vi "Robot Drive Manual.vi"(0 "Joystick0DevRef":T2={"Device"=enum."USB 1"}, 1 "RobotDriveDevRef":T4={"DevStatus"={"status"=FALSE, "code"=0, "source"=""}, "Motors[]"=[], "Square Inputs"=FALSE, "Max Output"=1.0}, 5 "Joystick1DevRef":T2={"Device"=enum."USB 1"}, 7 "Call Context":T1, 9 "Controller Mode":enum16{"X-Box Controller", "Joysticks"}(ring), 11 "Drive Mode":enum16{"Tank Drive", "Arcade Drive"}(ring), 12 "dt":dbl) -> (6 "Motor Values":dbl[](array[numeric]))   [LabVIEW 2016]
uses:
  <vilib>/Rock Robotics/WPI/RobotDrive/WPI_RobotDriveDevRef.ctl
  <vilib>/Rock Robotics/WPI/MotorControl/WPI_MotorControlDeviceRef.ctl
  <vilib>/Rock Robotics/WPI/MotorControl/WPI_MotorControlType.ctl
  <vilib>/Rock Robotics/SystemInterfaces/DIO/FPGA_DIOPWMChannel.ctl
  <vilib>/Rock Robotics/WPI/PWM/WPI_PWMDeadband.ctl
  <vilib>/Rock Robotics/WPI/Joystick/WPI_JoystickDevRef.ctl
  <vilib>/Rock Robotics/WPI/Joystick/WPI_JoystickDeviceEnum.ctl
  <vilib>/Rock Robotics/WPI/DriverStation/WPI_DriverStationDerivedRobotMode.ctl
  <vilib>/Rock Robotics/Network Tables/NT Read Boolean.vi
  Robot Global Data.vi
  <vilib>/Rock Robotics/Network Tables/NT Read Number.vi
  <vilib>/Rock Robotics/Network Tables/NT Write Numeric Array.vi
panel:
  in  "Axes (Joystick 1)":dbl[](array[numeric])
  in  "Axes (Joystick 0)":dbl[](array[numeric])
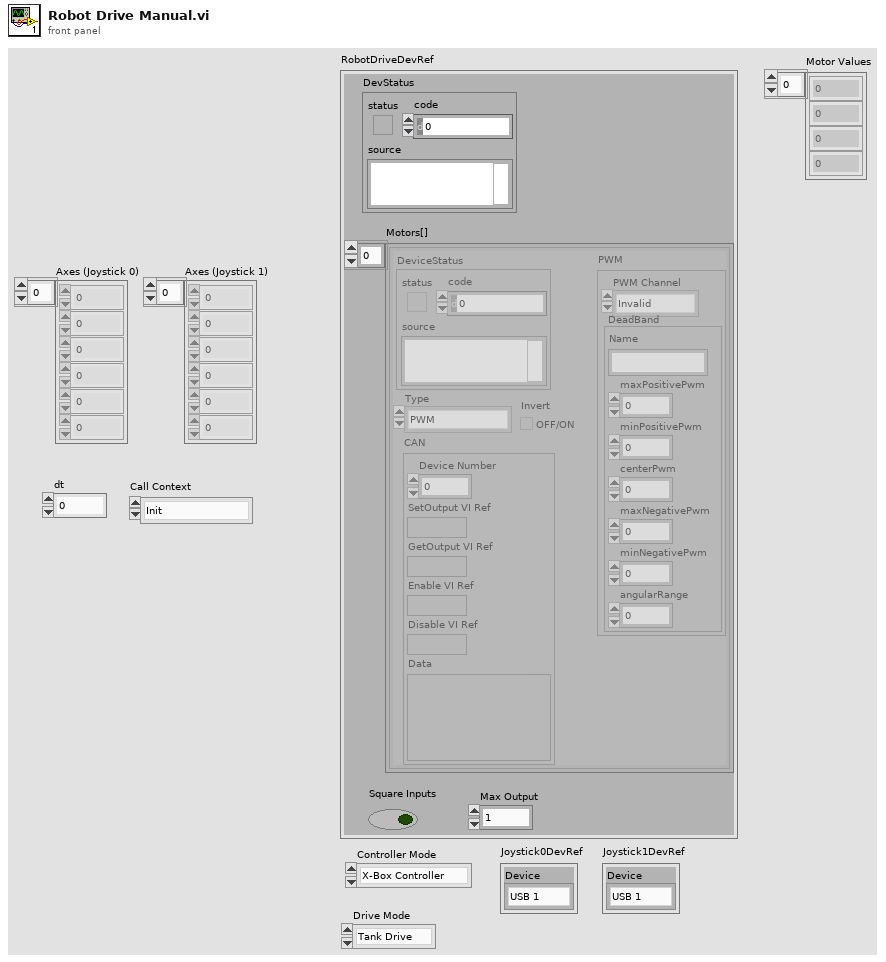
[diagram p1: front panel]
types:
  T1 = typedef "WPI_DriverStationDerivedRobotMode.ctl" = enum16{"Init", "Execute", "Stop"}
  T2 = typedef "WPI_JoystickDevRef.ctl" = cluster{"Device":T3}
  T3 = typedef "WPI_JoystickDeviceEnum.ctl" = enum16{"USB 0", "USB 1", "USB 2", "USB 3", "USB 4", "USB 5"}
  T4 = typedef "WPI_RobotDriveDevRef.ctl" = cluster{"DevStatus":errorcluster, "Motors[]":T5[], "Square Inputs":bool, "Max Output":dbl}
  T5 = typedef "WPI_MotorControlDeviceRef.ctl" = cluster{"DeviceStatus":errorcluster, "Type":T6, "PWM":cluster{"PWM Channel":T7, "DeadBand":T8}, "CAN":cluster{"Device Number":u8, "SetOutput VI Ref":variant, "GetOutput VI Ref":variant, "Enable VI Ref":variant, "Disable VI Ref":variant, "Data":variant}, "Invert":bool}
  T6 = typedef "WPI_MotorControlType.ctl" = enum16{"PWM", "CAN"}
  T7 = typedef "FPGA_DIOPWMChannel.ctl" = enum8{"PWM 0", "PWM 1", "PWM 2", "PWM 3", "PWM 4", "PWM 5", "PWM 6", "PWM 7", "PWM 8", "PWM 9", "PWM MXP 0", "PWM MXP 1", "PWM MXP 2", "PWM MXP 3", "PWM MXP 4", "PWM MXP 5", "PWM MXP 6", "PWM MXP 7", "PWM MXP 8", "PWM MXP 9", "Invalid"}
  T8 = typedef "WPI_PWMDeadband.ctl" = cluster{"Name":string, "maxPositivePwm":i32, "minPositivePwm":i32, "centerPwm":i32, "maxNegativePwm":i32, "minNegativePwm":i32, "angularRange":u16}
  T9 = cluster{"Current Gear":enum16{"Low", "High"}, "Gear Shift State":enum16{"Low", "Shifting", "High"}}
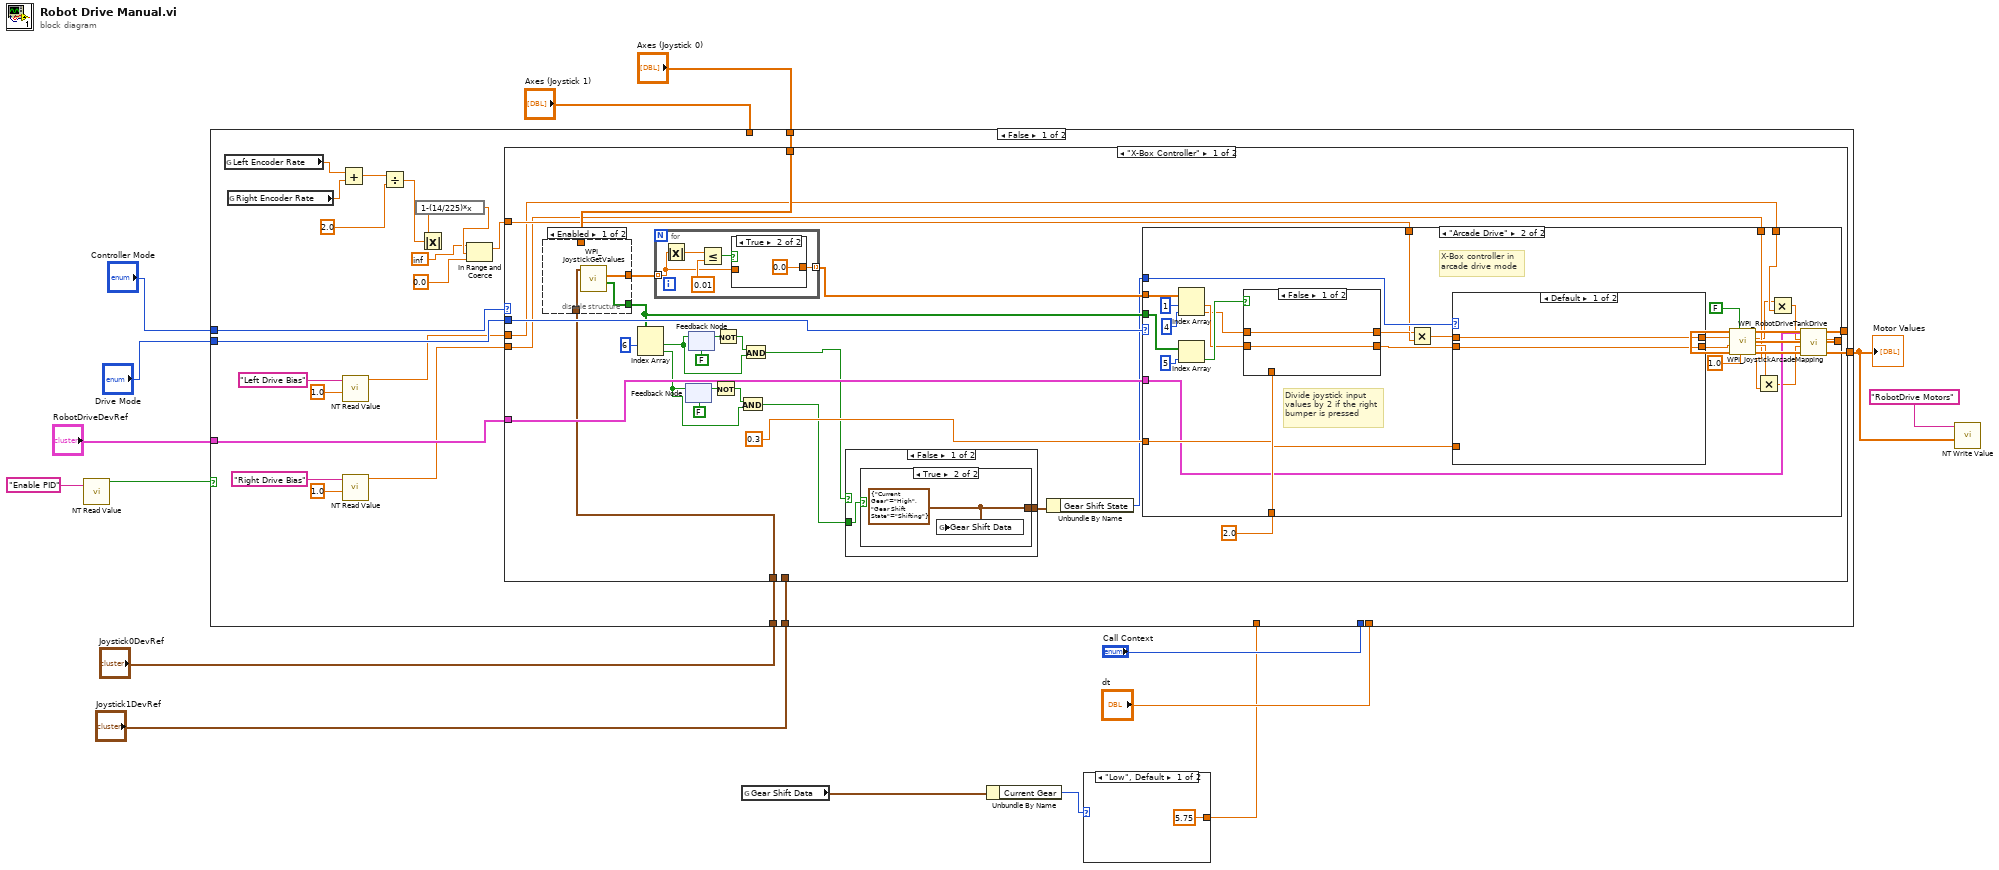
[diagram p0: block diagram]
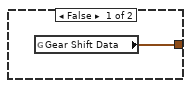
[diagram p2: hidden frame]
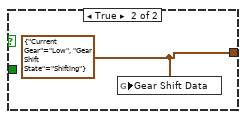
[diagram p3: hidden frame]
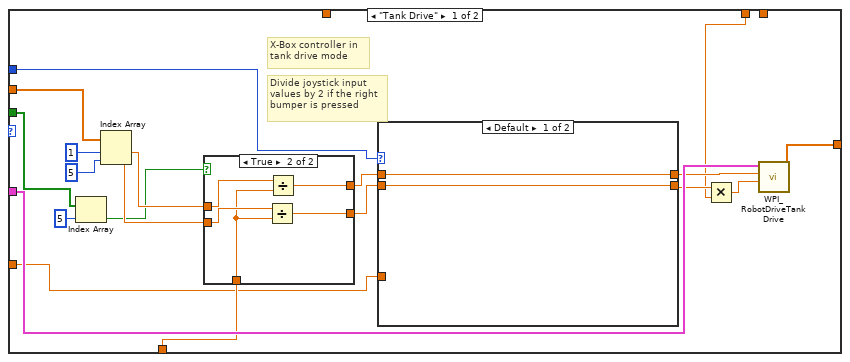
[diagram p4: hidden frame]
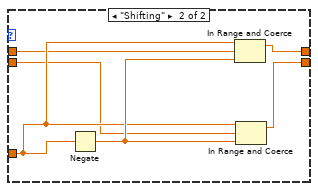
[diagram p5: hidden frame]
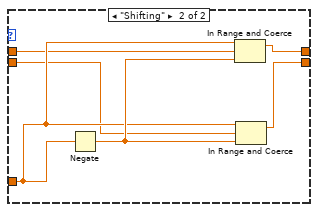
[diagram p7: hidden frame]
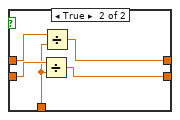
[diagram p8: hidden frame]
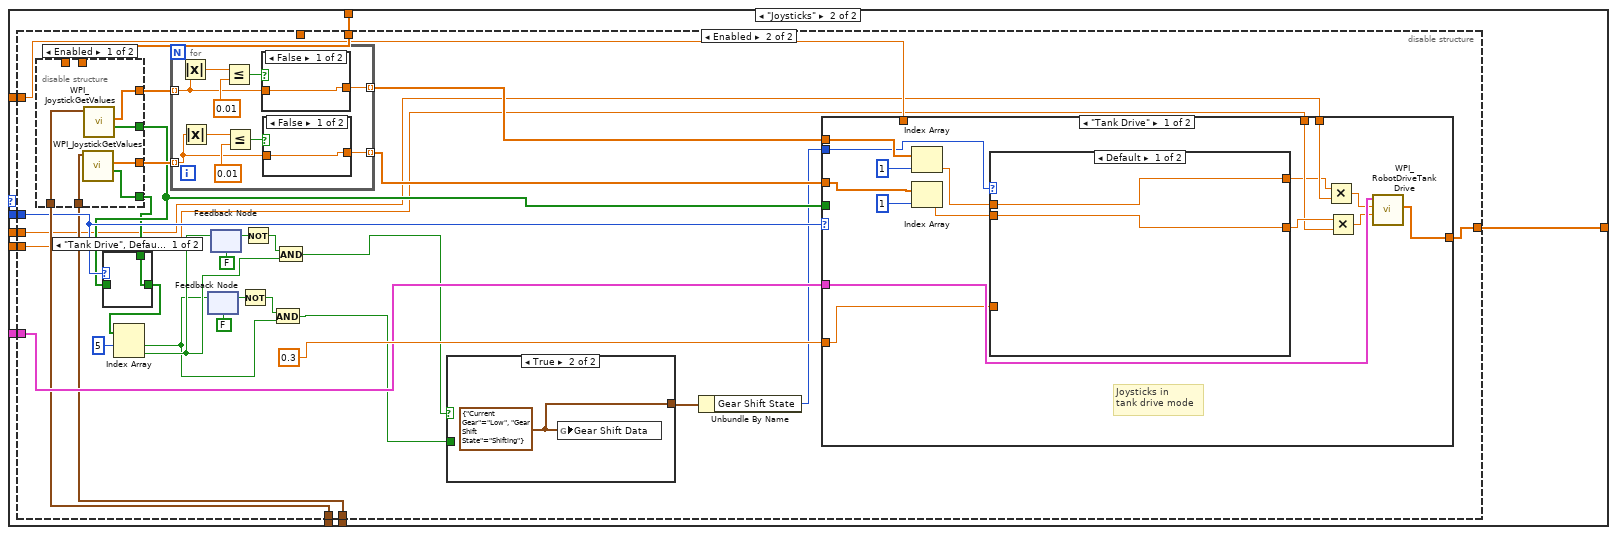
[diagram p11: hidden frame]
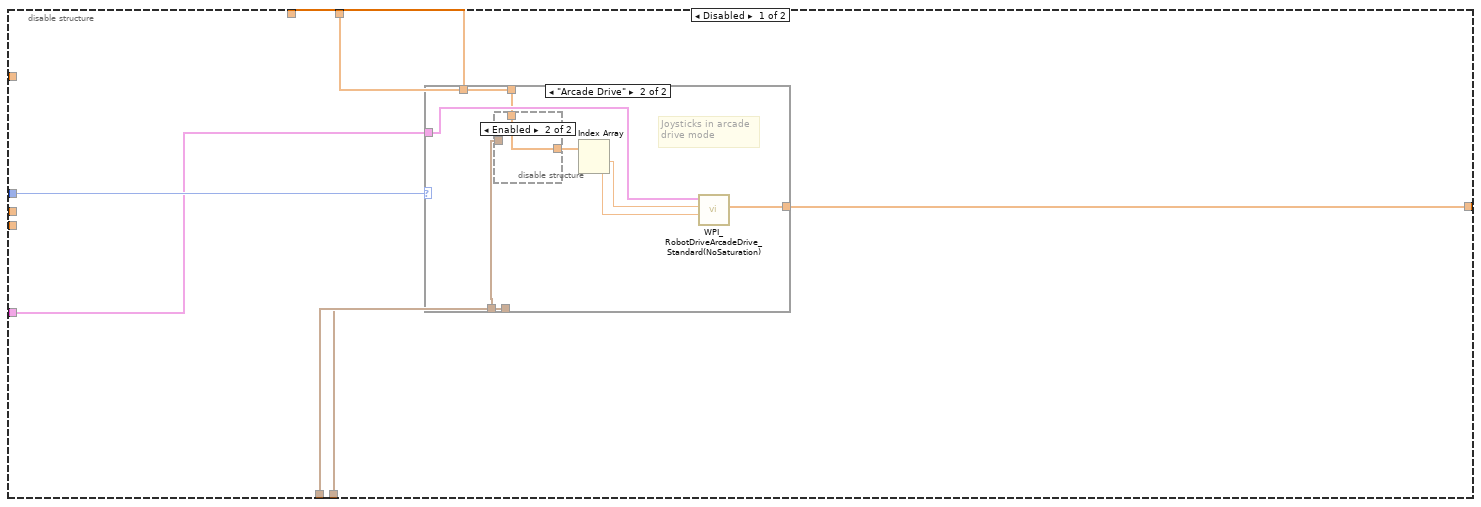
[diagram p12: hidden frame]
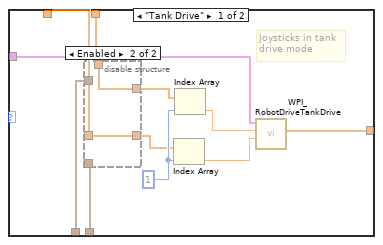
[diagram p13: hidden frame]
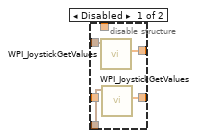
[diagram p14: hidden frame]
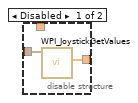
[diagram p15: hidden frame]
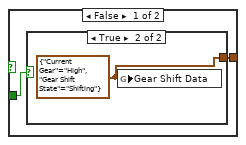
[diagram p16: hidden frame]
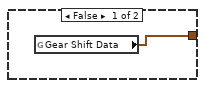
[diagram p17: hidden frame]
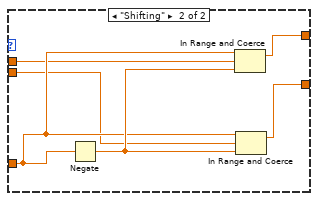
[diagram p18: hidden frame]
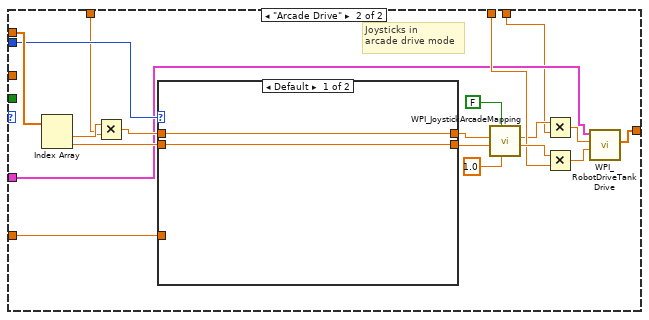
[diagram p19: hidden frame]
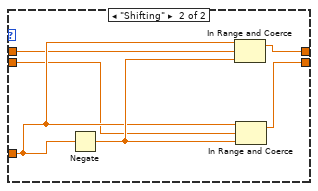
[diagram p20: hidden frame]
diagram:
  n1 = call-poly <vilib>:"NT Read Value.vi"("Name"="Enable PID") -> ("Boolean"=w1:bool)  [unwired: 9 in, 1 out]
  n2 = global read "Robot Global Data.vi" "Gear Shift Data"() -> (w5:T9)
  n3 = Unbundle By Name(w5) -> ("Current Gear"=w4:enum16{"Low", "High"})
  n4 = case shown="\"Low\", Default" w4 {
    tunnel: [5.75 14.75] -> w3
    frame "Low", Default {
    }
    frame "High" {
    }
  }
  n5 = case shown="False" w1 {
    tunnel: "Controller Mode" -> [w41 w324]
    tunnel: "Drive Mode" -> [w40 w323]
    tunnel: "RobotDriveDevRef" -> [w39 w322]
    tunnel: "Joystick0DevRef" -> [w38 w321]
    tunnel: "Joystick1DevRef" -> [w35 w320]
    tunnel: "Axes (Joystick 0)" -> [w37 w319]
    tunnel: "Axes (Joystick 1)" -> [_ w318]
    tunnel: [w36 w317] -> w8
    tunnel: "Call Context" -> [_ w316]
    tunnel: "dt" -> [_ w315]
    tunnel: w3 -> [_ w314]
    frame False {
      n6 = global read "Robot Global Data.vi" "Left Encoder Rate"() -> (w34:dbl)
      n7 = global read "Robot Global Data.vi" "Right Encoder Rate"() -> (w33:dbl)
      n8 = Add(x=w34, y=w33) -> (x+y=w32:dbl)
      n9 = call-poly <vilib>:"NT Read Value.vi"("Default Value"=1.0, "Name"="Left Drive Bias") -> ("Numeric"=w19:dbl)  [unwired: 8 in, 1 out]
      n10 = call-poly <vilib>:"NT Read Value.vi"("Default Value"=1.0, "Name"="Right Drive Bias") -> ("Numeric"=w23:dbl)  [unwired: 8 in, 1 out]
      n11 = Divide(x=w32, y=2.0) -> (x/y=w29:dbl)
      n12 = Absolute Value(x=w29) -> (abs(x)=w30:dbl)
      n13 = expression code="1-(14/225)*x"(w30) -> (w28:dbl)
      n14 = In Range and Coerce(upper limit=inf, x=w28, lower limit=0.0) -> (coerced(x)=w25:dbl)  [unwired: 1 out]
      n15 = case shown="\"X-Box Controller\"" w41 {
        tunnel: w40 -> [w67 w168]
        tunnel: w39 -> [w66 w166]
        tunnel: w38 -> [w64 w167]
        tunnel: [w65 w165] -> w36
        tunnel: w37 -> [w63 w164]
        tunnel: w35 -> [_ w163]
        tunnel: w25 -> [w44 w162]
        tunnel: w23 -> [w43 w161]
        tunnel: w19 -> [w42 w160]
        frame "X-Box Controller" {
          n16 = disable-structure shown="Enabled" {
            disable-tunnel: [w158 w159] -> w51
            disable-tunnel: w64 -> [w157 _]
            disable-tunnel: w63 -> [_ w159]
            disable-tunnel: [w156 _] -> w62
            frame Enabled {
              n17 = call <vilib>:"WPI_JoystickGetValues.vi"("JoystickDevRef"=w157) -> ("Buttons"=w156:bool[], "Axes"=w158:dbl[])  [unwired: 6 in, 3 out]
            }
            frame Disabled {
            }
          }
          n18 = Index Array(array=w62, index #1=6 ("index")) -> (element #1=w57:bool, element #2=w53:bool)  [unwired: 1 in]
          n19 = for {
            tunnel: w51 -> [w149] mode=indexing
            tunnel: [w150] -> w50 mode=indexing
            n20 = Absolute Value(x=w149) -> (abs(x)=w152:dbl)
            n21 = Less Or Equal?(x=w152, y=0.01) -> (x <= y?=w153:bool)
            n22 = case shown="True" w153 {
              tunnel: [w154 0.0] -> w150
              tunnel: w149 -> [w154 _]
              frame False {
              }
              frame True {
              }
            }
          }
          n23 = feedback #1(FALSE) -> (w55:bool)
          n24 = feedback-in #1(w53) -> ()
          n25 = feedback-in #2(w57) -> ()
          n26 = feedback #2(FALSE) -> (w59:bool)
          n27 = Not(x=w55) -> (.not. x?=w54:bool)
          n28 = Not(x=w59) -> (.not. x?=w58:bool)
          n29 = And(x=w54, y=w53) -> (x .and. y?=w47:bool)
          n30 = And(x=w58, y=w57) -> (x .and. y?=w48:bool)
          n31 = case shown="False" w48 {
            tunnel: w47 -> [w69 _]
            tunnel: [w68 w72] -> w46
            frame False {
              n32 = case shown="True" w69 {
                tunnel: [w70 w71] -> w68
                frame False {
                  n33 = global read "Robot Global Data.vi" "Gear Shift Data"() -> (w70:T9)
                }
                frame True {
                  w71 = T9 {"Current Gear"=enum."High", "Gear Shift State"=enum."Shifting"} ("Gear Shift Data")
                  n34 = global write "Robot Global Data.vi" "Gear Shift Data"(w71) -> ()
                }
              }
            }
            frame True {
              w72 = T9 {"Current Gear"=enum."Low", "Gear Shift State"=enum."Shifting"} ("Gear Shift Data")
              n35 = global write "Robot Global Data.vi" "Gear Shift Data"(w72) -> ()
            }
          }
          n36 = Unbundle By Name(w46) -> ("Gear Shift State"=w45:enum16{"Low", "Shifting", "High"})
          n37 = case shown="\"Arcade Drive\"" w67 {
            tunnel: w66 -> [w89 w113]
            tunnel: [w88 w114] -> w65
            tunnel: 2.0 -> [w85 w131]
            tunnel: w50 -> [w82 w130]
            tunnel: w62 -> [w81 w129]
            tunnel: 0.3 ("Left axis value") -> [w78 w126]
            tunnel: w45 -> [w77 w125]
            tunnel: w44 -> [_ w119]
            tunnel: w43 -> [w73 w110]
            tunnel: w42 -> [_ w108]
            frame "Tank Drive" {
              # "Divide joystick input\nvalues by 2 if the right\nbumper is pressed"
              # "X-Box controller in\ntank drive mode"
              n38 = Index Array(array=w81, index=5) -> (element=w83:bool)
              n39 = Index Array(array=w82, index #1=1 ("index"), index #2=5 ("index")) -> (element #1=w87:dbl, element #2=w86:dbl)
              n40 = case shown="True" w83 {
                tunnel: [w101 w106] -> w80
                tunnel: w87 -> [w101 w104]
                tunnel: [w100 w105] -> w79
                tunnel: w86 -> [w100 w103]
                tunnel: w85 -> [_ w102]
                frame False {
                }
                frame True {
                  n41 = Divide(x=w103, y=w102) -> (x/y=w105:dbl)
                  n42 = Divide(x=w104, y=w102) -> (x/y=w106:dbl)
                }
              }
              n43 = case shown="Default" w77 {
                tunnel: [w93 w95] -> w76
                tunnel: w80 -> [w93 w97]
                tunnel: [w92 w94] -> w74
                tunnel: w79 -> [w92 w96]
                tunnel: w78 -> [_ w98]
                frame Default {
                }
                frame "Shifting" {
                  n44 = Negate(x=w98) -> (-x=w99:dbl)
                  n45 = In Range and Coerce(upper limit=w98, x=w97, lower limit=w99) -> (coerced(x)=w95:dbl)  [unwired: 1 out]
                  n46 = In Range and Coerce(upper limit=w98, x=w96, lower limit=w99) -> (coerced(x)=w94:dbl)  [unwired: 1 out]
                }
              }
              n47 = Multiply(x=w74, y=w73) -> (x*y=w75:dbl)
              n48 = call <vilib>:"WPI_RobotDriveTankDrive.vi"("Right axis value"=w75, "Left axis value"=w76, "RobotDriveDevRef"=w89) -> ("Motor Values"=w88:dbl[])  [unwired: 6 in, 2 out]
            }
            frame "Arcade Drive" {
              # "Divide joystick input\nvalues by 2 if the right\nbumper is pressed"
              # "X-Box controller in\narcade drive mode"
              n49 = Index Array(array=w130, index #1=1 ("index"), index #2=4 ("index")) -> (element #1=w123:dbl, element #2=w122:dbl)
              n50 = Index Array(array=w129, index=5) -> (element=w132:bool)
              n51 = case shown="False" w132 {
                tunnel: [w143 w148] -> w120
                tunnel: w122 -> [w143 w146]
                tunnel: [w142 w147] -> w127
                tunnel: w123 -> [w142 w145]
                tunnel: w131 -> [_ w144]
                frame False {
                }
                frame True {
                  n52 = Divide(x=w145, y=w144) -> (x/y=w147:dbl)
                  n53 = Divide(x=w146, y=w144) -> (x/y=w148:dbl)
                }
              }
              n54 = Multiply(x=w119, y=w120) -> (x*y=w121:dbl)
              n55 = case shown="Default" w125 {
                tunnel: [w135 w137] -> w118
                tunnel: w121 -> [w135 w139]
                tunnel: [w134 w136] -> w117
                tunnel: w127 -> [w134 w138]
                tunnel: w126 -> [_ w140]
                frame Default {
                }
                frame "Shifting" {
                  n56 = Negate(x=w140) -> (-x=w141:dbl)
                  n57 = In Range and Coerce(upper limit=w140, x=w139, lower limit=w141) -> (coerced(x)=w137:dbl)  [unwired: 1 out]
                  n58 = In Range and Coerce(upper limit=w140, x=w138, lower limit=w141) -> (coerced(x)=w136:dbl)  [unwired: 1 out]
                }
              }
              n59 = call <vilib>:"WPI_JoystickArcadeMapping.vi"("Max Output"=1.0, "Square Inputs"=FALSE, "Y axis value"=w117, "X axis value"=w118) -> ("Right Motor Value"=w111:dbl, "Left Motor Value"=w107:dbl)  [unwired: 6 in]
              n60 = Multiply(x=w111, y=w110) -> (x*y=w112:dbl)
              n61 = Multiply(x=w107, y=w108) -> (x*y=w109:dbl)
              n62 = call <vilib>:"WPI_RobotDriveTankDrive.vi"("Right axis value"=w112, "Left axis value"=w109, "RobotDriveDevRef"=w113) -> ("Motor Values"=w114:dbl[])  [unwired: 6 in, 2 out]
            }
          }
        }
        frame "Joysticks" {
          n63 = disable-structure shown="Enabled" {
            disable-tunnel: w168 -> [w175 w217]
            disable-tunnel: w167 -> [w174 w220]
            disable-tunnel: w163 -> [w173 w210]
            disable-tunnel: w166 -> [w172 w222]
            disable-tunnel: [w171 w213] -> w165
            disable-tunnel: w164 -> [w170 w221]
            disable-tunnel: _ -> [w169 _]
            disable-tunnel: w162 -> [_ w205]
            disable-tunnel: w161 -> [_ w204]
            disable-tunnel: w160 -> [_ w203]
            frame Disabled {
              n64 = case shown="\"Arcade Drive\"" w175 {
                tunnel: w174 -> [w186 w195]
                tunnel: w173 -> [w185 _]
                tunnel: w172 -> [w181 w196]
                tunnel: [w178 w194] -> w171
                tunnel: w170 -> [w177 w193]
                tunnel: w169 -> [w176 _]
                frame "Tank Drive" {
                  w184 = 1
                  # "Joysticks in tank\ndrive mode"
                  n65 = disable-structure shown="Enabled" {
                    disable-tunnel: w186 -> [w190 _]
                    disable-tunnel: w185 -> [w189 _]
                    disable-tunnel: [w188 w192] -> w183
                    disable-tunnel: [w187 w191] -> w182
                    disable-tunnel: w177 -> [_ w192]
                    disable-tunnel: w176 -> [_ w191]
                    frame Disabled {
                      n66 = call <vilib>:"WPI_JoystickGetValues.vi"("JoystickDevRef"=w190) -> ("Axes"=w188:dbl[])  [unwired: 6 in, 4 out]
                      n67 = call <vilib>:"WPI_JoystickGetValues.vi"("JoystickDevRef"=w189) -> ("Axes"=w187:dbl[])  [unwired: 6 in, 4 out]
                    }
                    frame Enabled {
                    }
                  }
                  n68 = Index Array(array=w182, index=w184) -> (element=w179:dbl)
                  n69 = Index Array(array=w183, index=w184) -> (element=w180:dbl)
                  n70 = call <vilib>:"WPI_RobotDriveTankDrive.vi"("Right axis value"=w179, "Left axis value"=w180, "RobotDriveDevRef"=w181) -> ("Motor Values"=w178:dbl[])  [unwired: 6 in, 2 out]
                }
                frame "Arcade Drive" {
                  # "Joysticks in arcade\ndrive mode"
                  n71 = disable-structure shown="Enabled" {
                    disable-tunnel: [w201 w202] -> w199
                    disable-tunnel: w195 -> [w200 _]
                    disable-tunnel: w193 -> [_ w202]
                    frame Disabled {
                      n72 = call <vilib>:"WPI_JoystickGetValues.vi"("JoystickDevRef"=w200) -> ("Axes"=w201:dbl[])  [unwired: 6 in, 4 out]
                    }
                    frame Enabled {
                    }
                  }
                  n73 = Index Array(array=w199) -> (element #1=w198:dbl, element #2=w197:dbl)  [unwired: 2 in]
                  n74 = call <vilib>:"WPI_RobotDriveArcadeDrive_Standard(NoSaturation).vi"("Y axis value"=w197, "X axis value"=w198, "RobotDriveDevRef"=w196) -> ("Motor Values"=w194:dbl[])  [unwired: 1 in, 7 out]
                }
              }
            }
            frame Enabled {
              n75 = disable-structure shown="Enabled" {
                disable-tunnel: [w310 w311] -> w231
                disable-tunnel: w221 -> [_ w312]
                disable-tunnel: [w309 _] -> w214
                disable-tunnel: w220 -> [w308 _]
                disable-tunnel: [w307 w312] -> w219
                disable-tunnel: _ -> [_ w311]
                disable-tunnel: [w306 _] -> w216
                disable-tunnel: w210 -> [w305 _]
                frame Enabled {
                  n76 = call <vilib>:"WPI_JoystickGetValues.vi"("JoystickDevRef"=w305) -> ("Buttons"=w309:bool[], "Axes"=w310:dbl[])  [unwired: 6 in, 3 out]
                  n77 = call <vilib>:"WPI_JoystickGetValues.vi"("JoystickDevRef"=w308) -> ("Buttons"=w306:bool[], "Axes"=w307:dbl[])  [unwired: 6 in, 3 out]
                }
                frame Disabled {
                }
              }
              n78 = case shown="\"Tank Drive\", Default" w217 {
                tunnel: w216 -> [_ w290]
                tunnel: [w289 w290] -> w215
                tunnel: w214 -> [w289 _]
                frame "Tank Drive", Default {
                }
                frame "Arcade Drive" {
                }
              }
              n79 = Index Array(array=w215, index #1=5 ("index")) -> (element #1=w211:bool, element #2=w212:bool)  [unwired: 1 in]
              n80 = for {
                tunnel: w231 -> [w296] mode=indexing
                tunnel: [w297] -> w232 mode=indexing
                tunnel: w219 -> [w291] mode=indexing
                tunnel: [w292] -> w218 mode=indexing
                n81 = Absolute Value(x=w291) -> (abs(x)=w294:dbl)
                n82 = Absolute Value(x=w296) -> (abs(x)=w299:dbl)
                n83 = Less Or Equal?(x=w294, y=0.01) -> (x <= y?=w295:bool)
                n84 = Less Or Equal?(x=w299, y=0.01) -> (x <= y?=w300:bool)
                n85 = case shown="False" w295 {
                  tunnel: [w301 0.0] -> w292
                  tunnel: w291 -> [w301 _]
                  frame False {
                  }
                  frame True {
                  }
                }
                n86 = case shown="False" w300 {
                  tunnel: [w303 0.0] -> w297
                  tunnel: w296 -> [w303 _]
                  frame False {
                  }
                  frame True {
                  }
                }
              }
              n87 = feedback #3(FALSE) -> (w228:bool)
              n88 = feedback-in #3(w211) -> ()
              n89 = feedback #4(FALSE) -> (w225:bool)
              n90 = feedback-in #4(w212) -> ()
              n91 = Not(x=w228) -> (.not. x?=w229:bool)
              n92 = Not(x=w225) -> (.not. x?=w226:bool)
              n93 = And(x=w229, y=w211) -> (x .and. y?=w208:bool)
              n94 = And(x=w226, y=w212) -> (x .and. y?=w209:bool)
              n95 = case shown="True" w209 {
                tunnel: w208 -> [w234 _]
                tunnel: [w233 w237] -> w207
                frame False {
                  n96 = case shown="True" w234 {
                    tunnel: [w235 w236] -> w233
                    frame False {
                      n97 = global read "Robot Global Data.vi" "Gear Shift Data"() -> (w235:T9)
                    }
                    frame True {
                      w236 = T9 {"Current Gear"=enum."High", "Gear Shift State"=enum."Shifting"} ("Gear Shift Data")
                      n98 = global write "Robot Global Data.vi" "Gear Shift Data"(w236) -> ()
                    }
                  }
                }
                frame True {
                  w237 = T9 {"Current Gear"=enum."Low", "Gear Shift State"=enum."Shifting"} ("Gear Shift Data")
                  n99 = global write "Robot Global Data.vi" "Gear Shift Data"(w237) -> ()
                }
              }
              n100 = Unbundle By Name(w207) -> ("Gear Shift State"=w206:enum16{"Low", "Shifting", "High"})
              n101 = case shown="\"Tank Drive\"" w217 {
                tunnel: w222 -> [w252 w265]
                tunnel: [w251 w268] -> w213
                tunnel: w232 -> [w248 _]
                tunnel: w216 -> [_ _]
                tunnel: w218 -> [w249 w280]
                tunnel: 0.3 ("Left axis value") -> [w245 w278]
                tunnel: w206 -> [w244 w277]
                tunnel: w205 -> [_ w274]
                tunnel: w204 -> [w241 w266]
                tunnel: w203 -> [w239 w263]
                frame "Tank Drive" {
                  # "Joysticks in\ntank drive mode"
                  n102 = Index Array(array=w249, index=1) -> (element=w247:dbl)
                  n103 = Index Array(array=w248, index=1) -> (element=w246:dbl)
                  n104 = case shown="Default" w244 {
                    tunnel: [w255 w257] -> w238
                    tunnel: w247 -> [w255 w259]
                    tunnel: [w254 w256] -> w242
                    tunnel: w246 -> [w254 w258]
                    tunnel: w245 -> [_ w260]
                    frame Default {
                    }
                    frame "Shifting" {
                      n105 = Negate(x=w260) -> (-x=w261:dbl)
                      n106 = In Range and Coerce(upper limit=w260, x=w259, lower limit=w261) -> (coerced(x)=w257:dbl)  [unwired: 1 out]
                      n107 = In Range and Coerce(upper limit=w260, x=w258, lower limit=w261) -> (coerced(x)=w256:dbl)  [unwired: 1 out]
                    }
                  }
                  n108 = Multiply(x=w238, y=w239) -> (x*y=w240:dbl)
                  n109 = Multiply(x=w242, y=w241) -> (x*y=w243:dbl)
                  n110 = call <vilib>:"WPI_RobotDriveTankDrive.vi"("Right axis value"=w243, "Left axis value"=w240, "RobotDriveDevRef"=w252) -> ("Motor Values"=w251:dbl[])  [unwired: 6 in, 2 out]
                }
                frame "Arcade Drive" {
                  # "Joysticks in\narcade drive mode"
                  n111 = Index Array(array=w280) -> (element #1=w275:dbl, element #2=w279:dbl)  [unwired: 2 in]
                  n112 = Multiply(x=w275, y=w274) -> (x*y=w276:dbl)
                  n113 = case shown="Default" w277 {
                    tunnel: [w282 w284] -> w273
                    tunnel: w276 -> [w282 w286]
                    tunnel: [w281 w283] -> w272
                    tunnel: w279 -> [w281 w285]
                    tunnel: w278 -> [_ w287]
                    frame Default {
                    }
                    frame "Shifting" {
                      n114 = Negate(x=w287) -> (-x=w288:dbl)
                      n115 = In Range and Coerce(upper limit=w287, x=w286, lower limit=w288) -> (coerced(x)=w284:dbl)  [unwired: 1 out]
                      n116 = In Range and Coerce(upper limit=w287, x=w285, lower limit=w288) -> (coerced(x)=w283:dbl)  [unwired: 1 out]
                    }
                  }
                  n117 = call <vilib>:"WPI_JoystickArcadeMapping.vi"("Max Output"=1.0, "Square Inputs"=FALSE, "Y axis value"=w272, "X axis value"=w273) -> ("Right Motor Value"=w269:dbl, "Left Motor Value"=w264:dbl)  [unwired: 6 in]
                  n118 = Multiply(x=w264, y=w263) -> (x*y=w262:dbl)
                  n119 = Multiply(x=w269, y=w266) -> (x*y=w267:dbl)
                  n120 = call <vilib>:"WPI_RobotDriveTankDrive.vi"("Right axis value"=w267, "Left axis value"=w262, "RobotDriveDevRef"=w265) -> ("Motor Values"=w268:dbl[])  [unwired: 6 in, 2 out]
                }
              }
            }
          }
        }
      }
    }
    frame True {
      n121 = case shown="\"X-Box Controller\"" w324 {
        tunnel: w323 -> [w349 w479]
        tunnel: w322 -> [w348 w476]
        tunnel: w321 -> [w343 w478]
        tunnel: [w347 w475] -> w317
        tunnel: w320 -> [_ w477]
        tunnel: w319 -> [w342 w474]
        tunnel: w318 -> [_ w473]
        tunnel: w316 -> [w346 w471]
        tunnel: w315 -> [w345 w472]
        tunnel: w314 -> [w344 w470]
        tunnel: 1.0 -> [w325 w469]
        frame "X-Box Controller" {
          n122 = disable-structure shown="Enabled" {
            disable-tunnel: [w467 w468] -> w327
            disable-tunnel: w343 -> [w466 _]
            disable-tunnel: w342 -> [_ w468]
            disable-tunnel: [w465 _] -> w341
            frame Enabled {
              n123 = call <vilib>:"WPI_JoystickGetValues.vi"("JoystickDevRef"=w466) -> ("Buttons"=w465:bool[], "Axes"=w467:dbl[])  [unwired: 6 in, 3 out]
            }
            frame Disabled {
            }
          }
          n124 = Index Array(array=w341, index #1=6 ("index")) -> (element #1=w336:bool, element #2=w332:bool)  [unwired: 1 in]
          n125 = for {
            tunnel: w327 -> [w350] mode=indexing
            tunnel: [w351] -> w326 mode=indexing
            n126 = Absolute Value(x=w350) -> (abs(x)=w353:dbl)
            n127 = Less Or Equal?(x=w353, y=0.01) -> (x <= y?=w354:bool)
            n128 = case shown="True" w354 {
              tunnel: [w355 0.0] -> w351
              tunnel: w350 -> [w355 _]
              frame False {
              }
              frame True {
              }
            }
          }
          n129 = feedback #5(FALSE) -> (w334:bool)
          n130 = feedback-in #5(w332) -> ()
          n131 = feedback-in #6(w336) -> ()
          n132 = feedback #6(FALSE) -> (w338:bool)
          n133 = Not(x=w334) -> (.not. x?=w333:bool)
          n134 = Not(x=w338) -> (.not. x?=w337:bool)
          n135 = And(x=w333, y=w332) -> (x .and. y?=w329:bool)
          n136 = And(x=w337, y=w336) -> (x .and. y?=w330:bool)
          n137 = Or(x=w330, y=w329) -> (x .or. y?=w331:bool)
          n138 = case shown="False" w331 {
            tunnel: w349 -> [w368 _]
            tunnel: w348 -> [w367 w459]
            tunnel: [w366 w458] -> w347
            tunnel: w346 -> [w365 _]
            tunnel: w345 -> [w364 _]
            tunnel: w344 -> [w363 _]
            tunnel: w326 -> [w362 _]
            tunnel: w341 -> [w361 _]
            tunnel: w330 -> [_ w461]
            tunnel: w329 -> [_ w460]
            tunnel: 0.3 ("Left axis value") -> [w358 w454]
            tunnel: w325 -> [w357 _]
            frame False {
              n139 = global read "Robot Global Data.vi" "Gear Shift Data"() -> (w360:T9)
              n140 = Unbundle By Name(w360) -> ("Gear Shift State"=w359:enum16{"Low", "Shifting", "High"})
              n141 = case shown="Default" w359 {
                tunnel: w368 -> [w378 _]
                tunnel: w367 -> [w377 w451]
                tunnel: [w376 w450] -> w366
                tunnel: w365 -> [w374 _]
                tunnel: w364 -> [w373 _]
                tunnel: w363 -> [w372 _]
                tunnel: w362 -> [w371 _]
                tunnel: w361 -> [w370 _]
                tunnel: w358 -> [_ w447]
                tunnel: w357 -> [w369 _]
                frame Default {
                  n142 = case shown="\"Arcade Drive\"" w378 {
                    tunnel: w377 -> [w398 w428]
                    tunnel: [w397 w429] -> w376
                    tunnel: 2.0 -> [w396 w434]
                    tunnel: w374 -> [w393 w431]
                    tunnel: w373 -> [w392 w430]
                    tunnel: w372 -> [w391 w424]
                    tunnel: w371 -> [w386 w427]
                    tunnel: w370 -> [w385 w426]
                    tunnel: w369 -> [_ w425]
                    frame "Tank Drive" {
                      # "Divide joystick input\nvalues by 2 if the right\nbumper is pressed"
                      # "X-Box controller in\ntank drive mode"
                      n143 = Index Array(array=w385, index=5) -> (element=w394:bool)
                      n144 = Index Array(array=w386, index #1=1 ("index"), index #2=5 ("index")) -> (element #1=w380:dbl, element #2=w379:dbl)
                      n145 = case shown="True" w394 {
                        tunnel: [w402 w407] -> w390
                        tunnel: w380 -> [w402 w405]
                        tunnel: [w401 w406] -> w389
                        tunnel: w379 -> [w401 w404]
                        tunnel: w396 -> [_ w403]
                        frame False {
                        }
                        frame True {
                          n146 = Divide(x=w404, y=w403) -> (x/y=w406:dbl)
                          n147 = Divide(x=w405, y=w403) -> (x/y=w407:dbl)
                        }
                      }
                      n148 = Multiply(x=w390, y=w391) -> (x*y=w384:dbl)
                      n149 = Multiply(x=w389, y=w391) -> (x*y=w382:dbl)
                      n150 = Negate(x=w384) -> (-x=w383:dbl)
                      n151 = Negate(x=w382) -> (-x=w381:dbl)
                      n152 = call "PID Robot Drive.vi"("dt"=w392, "Right RPS"=w381, "Left RPS"=w383, "Robot Mode Call Context"=w393) -> ("Right Throttle"=w387:dbl, "Left Throttle"=w388:dbl)  [unwired: 6 in]
                      n153 = call <vilib>:"WPI_RobotDriveTankDrive.vi"("Right axis value"=w387, "Left axis value"=w388, "RobotDriveDevRef"=w398) -> ("Motor Values"=w397:dbl[])  [unwired: 6 in, 2 out]
                    }
                    frame "Arcade Drive" {
                      # "Divide joystick input\nvalues by 2 if the right\nbumper is pressed"
                      # "X-Box controller in\narcade drive mode"
                      n154 = Index Array(array=w427, index #1=1 ("index"), index #2=4 ("index")) -> (element #1=w408:dbl, element #2=w409:dbl)
                      n155 = Index Array(array=w426, index=5) -> (element=w435:bool)
                      n156 = Multiply(x=w409, y=w425) -> (x*y=w411:dbl)
                      n157 = Divide(x=w411, y=w424) -> (x/y=w423:dbl)
                      n158 = case shown="False" w435 {
                        tunnel: [w438 w443] -> w433
                        tunnel: w423 -> [w438 w441]
                        tunnel: [w437 w442] -> w432
                        tunnel: w408 -> [w437 w440]
                        tunnel: w434 -> [_ w439]
                        frame False {
                        }
                        frame True {
                          n159 = Divide(x=w440, y=w439) -> (x/y=w442:dbl)
                          n160 = Divide(x=w441, y=w439) -> (x/y=w443:dbl)
                        }
                      }
                      n161 = call <vilib>:"WPI_JoystickArcadeMapping.vi"("Max Output"=1.0, "Square Inputs"=FALSE, "Y axis value"=w432, "X axis value"=w433) -> ("Right Motor Value"=w418:dbl, "Left Motor Value"=w419:dbl)  [unwired: 6 in]
                      n162 = Multiply(x=w419, y=w424) -> (x*y=w414:dbl)
                      n163 = Multiply(x=w418, y=w424) -> (x*y=w415:dbl)
                      n164 = Negate(x=w414) -> (-x=w413:dbl)
                      n165 = Negate(x=w415) -> (-x=w412:dbl)
                      n166 = call "PID Robot Drive.vi"("dt"=w430, "Right RPS"=w412, "Left RPS"=w413, "Robot Mode Call Context"=w431) -> ("Right Throttle"=w416:dbl, "Left Throttle"=w417:dbl)  [unwired: 6 in]
                      n167 = call <vilib>:"WPI_RobotDriveTankDrive.vi"("Right axis value"=w416, "Left axis value"=w417, "RobotDriveDevRef"=w428) -> ("Motor Values"=w429:dbl[])  [unwired: 6 in, 2 out]
                    }
                  }
                }
                frame "Shifting" {
                  n168 = global read "Robot Global Data.vi" "PID Left Motor Throttle"() -> (w449:dbl)
                  n169 = global read "Robot Global Data.vi" "PID Right Motor Throttle"() -> (w448:dbl)
                  n170 = Negate(x=w447) -> (-x=w446:dbl)
                  n171 = In Range and Coerce(upper limit=w447, x=w449, lower limit=w446) -> (coerced(x)=w445:dbl)  [unwired: 1 out]
                  n172 = In Range and Coerce(upper limit=w447, x=w448, lower limit=w446) -> (coerced(x)=w444:dbl)  [unwired: 1 out]
                  n173 = call <vilib>:"WPI_RobotDriveTankDrive.vi"("Right axis value"=w444, "Left axis value"=w445, "RobotDriveDevRef"=w451) -> ("Motor Values"=w450:dbl[])  [unwired: 6 in, 2 out]
                }
              }
            }
            frame True {
              n174 = case shown="False" w461 {
                tunnel: w460 -> [w462 _]
                frame False {
                  n175 = case shown="True" w462 {
                    frame False {
                    }
                    frame True {
                      n176 = global write "Robot Global Data.vi" "Gear Shift Data"(T9 {"Current Gear"=enum."High", "Gear Shift State"=enum."Shifting"} ("Gear Shift Data")) -> ()
                    }
                  }
                }
                frame True {
                  n177 = global write "Robot Global Data.vi" "Gear Shift Data"(T9 {"Current Gear"=enum."Low", "Gear Shift State"=enum."Shifting"} ("Gear Shift Data")) -> ()
                }
              }
              n178 = global read "Robot Global Data.vi" "PID Left Motor Throttle"() -> (w457:dbl)
              n179 = global read "Robot Global Data.vi" "PID Right Motor Throttle"() -> (w456:dbl)
              n180 = Negate(x=w454) -> (-x=w455:dbl)
              n181 = In Range and Coerce(upper limit=w454, x=w457, lower limit=w455) -> (coerced(x)=w453:dbl)  [unwired: 1 out]
              n182 = In Range and Coerce(upper limit=w454, x=w456, lower limit=w455) -> (coerced(x)=w452:dbl)  [unwired: 1 out]
              n183 = call <vilib>:"WPI_RobotDriveTankDrive.vi"("Right axis value"=w452, "Left axis value"=w453, "RobotDriveDevRef"=w459) -> ("Motor Values"=w458:dbl[])  [unwired: 6 in, 2 out]
            }
          }
        }
        frame "Joysticks" {
          n184 = disable-structure shown="Enabled" {
            disable-tunnel: w479 -> [w486 w521]
            disable-tunnel: w478 -> [w485 w528]
            disable-tunnel: w477 -> [w484 w529]
            disable-tunnel: w476 -> [w483 w531]
            disable-tunnel: [w482 w517] -> w475
            disable-tunnel: w474 -> [w481 w530]
            disable-tunnel: w473 -> [w480 w526]
            disable-tunnel: w472 -> [_ w525]
            disable-tunnel: w471 -> [_ w524]
            disable-tunnel: w470 -> [_ w523]
            disable-tunnel: w469 -> [_ w514]
            frame Disabled {
              n185 = case shown="\"Arcade Drive\"" w486 {
                tunnel: w485 -> [w497 w506]
                tunnel: w484 -> [w496 _]
                tunnel: w483 -> [w492 w507]
                tunnel: [w489 w505] -> w482
                tunnel: w481 -> [w488 w504]
                tunnel: w480 -> [w487 _]
                frame "Tank Drive" {
                  w495 = 1
                  # "Joysticks in tank\ndrive mode"
                  n186 = disable-structure shown="Enabled" {
                    disable-tunnel: w497 -> [w501 _]
                    disable-tunnel: w496 -> [w500 _]
                    disable-tunnel: [w499 w503] -> w494
                    disable-tunnel: [w498 w502] -> w493
                    disable-tunnel: w488 -> [_ w503]
                    disable-tunnel: w487 -> [_ w502]
                    frame Disabled {
                      n187 = call <vilib>:"WPI_JoystickGetValues.vi"("JoystickDevRef"=w501) -> ("Axes"=w499:dbl[])  [unwired: 6 in, 4 out]
                      n188 = call <vilib>:"WPI_JoystickGetValues.vi"("JoystickDevRef"=w500) -> ("Axes"=w498:dbl[])  [unwired: 6 in, 4 out]
                    }
                    frame Enabled {
                    }
                  }
                  n189 = Index Array(array=w493, index=w495) -> (element=w490:dbl)
                  n190 = Index Array(array=w494, index=w495) -> (element=w491:dbl)
                  n191 = call <vilib>:"WPI_RobotDriveTankDrive.vi"("Right axis value"=w490, "Left axis value"=w491, "RobotDriveDevRef"=w492) -> ("Motor Values"=w489:dbl[])  [unwired: 6 in, 2 out]
                }
                frame "Arcade Drive" {
                  # "Joysticks in arcade\ndrive mode"
                  n192 = disable-structure shown="Enabled" {
                    disable-tunnel: [w512 w513] -> w510
                    disable-tunnel: w506 -> [w511 _]
                    disable-tunnel: w504 -> [_ w513]
                    frame Disabled {
                      n193 = call <vilib>:"WPI_JoystickGetValues.vi"("JoystickDevRef"=w511) -> ("Axes"=w512:dbl[])  [unwired: 6 in, 4 out]
                    }
                    frame Enabled {
                    }
                  }
                  n194 = Index Array(array=w510) -> (element #1=w509:dbl, element #2=w508:dbl)  [unwired: 2 in]
                  n195 = call <vilib>:"WPI_RobotDriveArcadeDrive_Standard(NoSaturation).vi"("Y axis value"=w508, "X axis value"=w509, "RobotDriveDevRef"=w507) -> ("Motor Values"=w505:dbl[])  [unwired: 1 in, 7 out]
                }
              }
            }
            frame Enabled {
              n196 = disable-structure shown="Enabled" {
                disable-tunnel: [w646 w647] -> w543
                disable-tunnel: w529 -> [w645 _]
                disable-tunnel: w530 -> [_ w648]
                disable-tunnel: [w644 _] -> w518
                disable-tunnel: w528 -> [w643 _]
                disable-tunnel: [w642 w648] -> w527
                disable-tunnel: w526 -> [_ w647]
                disable-tunnel: [w641 _] -> w520
                frame Enabled {
                  n197 = call <vilib>:"WPI_JoystickGetValues.vi"("JoystickDevRef"=w645) -> ("Buttons"=w644:bool[], "Axes"=w646:dbl[])  [unwired: 6 in, 3 out]
                  n198 = call <vilib>:"WPI_JoystickGetValues.vi"("JoystickDevRef"=w643) -> ("Buttons"=w641:bool[], "Axes"=w642:dbl[])  [unwired: 6 in, 3 out]
                }
                frame Disabled {
                }
              }
              n199 = case shown="\"Tank Drive\", Default" w521 {
                tunnel: w520 -> [_ w546]
                tunnel: [w545 w546] -> w519
                tunnel: w518 -> [w545 _]
                frame "Tank Drive", Default {
                }
                frame "Arcade Drive" {
                }
              }
              n200 = Index Array(array=w519, index #1=5 ("index")) -> (element #1=w515:bool, element #2=w516:bool)  [unwired: 1 in]
              n201 = for {
                tunnel: w543 -> [w552] mode=indexing
                tunnel: [w553] -> w544 mode=indexing
                tunnel: w527 -> [w547] mode=indexing
                tunnel: [w548] -> w522 mode=indexing
                n202 = Absolute Value(x=w547) -> (abs(x)=w550:dbl)
                n203 = Absolute Value(x=w552) -> (abs(x)=w555:dbl)
                n204 = Less Or Equal?(x=w550, y=0.01) -> (x <= y?=w551:bool)
                n205 = Less Or Equal?(x=w555, y=0.01) -> (x <= y?=w556:bool)
                n206 = case shown="False" w551 {
                  tunnel: [w557 0.0] -> w548
                  tunnel: w547 -> [w557 _]
                  frame False {
                  }
                  frame True {
                  }
                }
                n207 = case shown="False" w556 {
                  tunnel: [w559 0.0] -> w553
                  tunnel: w552 -> [w559 _]
                  frame False {
                  }
                  frame True {
                  }
                }
              }
              n208 = feedback #7(FALSE) -> (w537:bool)
              n209 = feedback-in #7(w515) -> ()
              n210 = feedback #8(FALSE) -> (w534:bool)
              n211 = feedback-in #8(w516) -> ()
              n212 = Not(x=w537) -> (.not. x?=w538:bool)
              n213 = Not(x=w534) -> (.not. x?=w535:bool)
              n214 = And(x=w538, y=w515) -> (x .and. y?=w541:bool)
              n215 = And(x=w535, y=w516) -> (x .and. y?=w540:bool)
              n216 = Or(x=w540, y=w541) -> (x .or. y?=w539:bool)
              n217 = case shown="False" w539 {
                tunnel: w521 -> [w573 _]
                tunnel: w531 -> [w572 w635]
                tunnel: [w571 w634] -> w517
                tunnel: w524 -> [w570 _]
                tunnel: w525 -> [w569 _]
                tunnel: w523 -> [w568 _]
                tunnel: w544 -> [w567 _]
                tunnel: w540 -> [_ w637]
                tunnel: w541 -> [_ w636]
                tunnel: 0.3 ("Left axis value") -> [w564 w630]
                tunnel: w520 -> [w563 _]
                tunnel: w518 -> [_ _]
                tunnel: w522 -> [w562 _]
                tunnel: w514 -> [w561 _]
                frame False {
                  n218 = global read "Robot Global Data.vi" "Gear Shift Data"() -> (w566:T9)
                  n219 = Unbundle By Name(w566) -> ("Gear Shift State"=w565:enum16{"Low", "Shifting", "High"})
                  n220 = case shown="Default" w565 {
                    tunnel: w573 -> [w583 _]
                    tunnel: w572 -> [w582 w627]
                    tunnel: [w581 w626] -> w571
                    tunnel: w570 -> [w580 _]
                    tunnel: w569 -> [w579 _]
                    tunnel: w568 -> [w578 _]
                    tunnel: w567 -> [w577 _]
                    tunnel: w563 -> [w576 _]
                    tunnel: w564 -> [_ w623]
                    tunnel: w562 -> [w575 _]
                    tunnel: w561 -> [w574 _]
                    frame Default {
                      n221 = case shown="\"Arcade Drive\"" w583 {
                        tunnel: w582 -> [w599 w610]
                        tunnel: [w598 w611] -> w581
                        tunnel: w580 -> [w597 w615]
                        tunnel: w579 -> [w596 w614]
                        tunnel: w578 -> [w595 w601]
                        tunnel: w577 -> [w586 _]
                        tunnel: w576 -> [_ _]
                        tunnel: w575 -> [w587 w606]
                        tunnel: w574 -> [_ w602]
                        frame "Tank Drive" {
                          # "Joysticks in\ntank drive mode"
                          n222 = Index Array(array=w587, index=1) -> (element=w585:dbl)
                          n223 = Index Array(array=w586, index=1) -> (element=w584:dbl)
                          n224 = Multiply(x=w585, y=w595) -> (x*y=w592:dbl)
                          n225 = Multiply(x=w584, y=w595) -> (x*y=w590:dbl)
                          n226 = Negate(x=w592) -> (-x=w591:dbl)
                          n227 = Negate(x=w590) -> (-x=w589:dbl)
                          n228 = call "PID Robot Drive.vi"("dt"=w596, "Right RPS"=w589, "Left RPS"=w591, "Robot Mode Call Context"=w597) -> ("Right Throttle"=w593:dbl, "Left Throttle"=w594:dbl)  [unwired: 6 in]
                          n229 = call <vilib>:"WPI_RobotDriveTankDrive.vi"("Right axis value"=w593, "Left axis value"=w594, "RobotDriveDevRef"=w599) -> ("Motor Values"=w598:dbl[])  [unwired: 6 in, 2 out]
                        }
                        frame "Arcade Drive" {
                          # "Joysticks in\narcade drive mode"
                          n230 = Index Array(array=w606) -> (element #1=w603:dbl, element #2=w607:dbl)  [unwired: 2 in]
                          n231 = Multiply(x=w603, y=w602) -> (x*y=w605:dbl)
                          n232 = Divide(x=w605, y=w601) -> (x/y=w604:dbl)
                          n233 = call <vilib>:"WPI_JoystickArcadeMapping.vi"("Max Output"=1.0, "Square Inputs"=FALSE, "Y axis value"=w607, "X axis value"=w604) -> ("Right Motor Value"=w616:dbl, "Left Motor Value"=w617:dbl)  [unwired: 6 in]
                          n234 = Multiply(x=w617, y=w601) -> (x*y=w613:dbl)
                          n235 = Multiply(x=w616, y=w601) -> (x*y=w612:dbl)
                          n236 = call "PID Robot Drive.vi"("dt"=w614, "Right RPS"=w612, "Left RPS"=w613, "Robot Mode Call Context"=w615) -> ("Right Throttle"=w608:dbl, "Left Throttle"=w609:dbl)  [unwired: 6 in]
                          n237 = call <vilib>:"WPI_RobotDriveTankDrive.vi"("Right axis value"=w608, "Left axis value"=w609, "RobotDriveDevRef"=w610) -> ("Motor Values"=w611:dbl[])  [unwired: 6 in, 2 out]
                        }
                      }
                    }
                    frame "Shifting" {
                      n238 = global read "Robot Global Data.vi" "PID Left Motor Throttle"() -> (w625:dbl)
                      n239 = global read "Robot Global Data.vi" "PID Right Motor Throttle"() -> (w624:dbl)
                      n240 = Negate(x=w623) -> (-x=w622:dbl)
                      n241 = In Range and Coerce(upper limit=w623, x=w625, lower limit=w622) -> (coerced(x)=w621:dbl)  [unwired: 1 out]
                      n242 = In Range and Coerce(upper limit=w623, x=w624, lower limit=w622) -> (coerced(x)=w620:dbl)  [unwired: 1 out]
                      n243 = call <vilib>:"WPI_RobotDriveTankDrive.vi"("Right axis value"=w620, "Left axis value"=w621, "RobotDriveDevRef"=w627) -> ("Motor Values"=w626:dbl[])  [unwired: 6 in, 2 out]
                    }
                  }
                }
                frame True {
                  n244 = case shown="True" w637 {
                    tunnel: w636 -> [w638 _]
                    frame False {
                      n245 = case shown="True" w638 {
                        frame False {
                        }
                        frame True {
                          n246 = global write "Robot Global Data.vi" "Gear Shift Data"(T9 {"Current Gear"=enum."High", "Gear Shift State"=enum."Shifting"} ("Gear Shift Data")) -> ()
                        }
                      }
                    }
                    frame True {
                      n247 = global write "Robot Global Data.vi" "Gear Shift Data"(T9 {"Current Gear"=enum."Low", "Gear Shift State"=enum."Shifting"} ("Gear Shift Data")) -> ()
                    }
                  }
                  n248 = global read "Robot Global Data.vi" "PID Left Motor Throttle"() -> (w633:dbl)
                  n249 = global read "Robot Global Data.vi" "PID Right Motor Throttle"() -> (w632:dbl)
                  n250 = Negate(x=w630) -> (-x=w631:dbl)
                  n251 = In Range and Coerce(upper limit=w630, x=w633, lower limit=w631) -> (coerced(x)=w629:dbl)  [unwired: 1 out]
                  n252 = In Range and Coerce(upper limit=w630, x=w632, lower limit=w631) -> (coerced(x)=w628:dbl)  [unwired: 1 out]
                  n253 = call <vilib>:"WPI_RobotDriveTankDrive.vi"("Right axis value"=w628, "Left axis value"=w629, "RobotDriveDevRef"=w635) -> ("Motor Values"=w634:dbl[])  [unwired: 6 in, 2 out]
                }
              }
            }
          }
        }
      }
    }
  }
  "Motor Values" <- w8
  n254 = call-poly <vilib>:"NT Write Value.vi"("Numeric Array"=w8, "Name"="RobotDrive Motors") -> ()  [unwired: 9 in, 1 out]
